vi "Refresh Modules.vi"(8 "error in (no error)":errorcluster, 11 "target address (localhost)":string="localhost") -> (0 "error out":errorcluster)   [LabVIEW 2020]
doc: "Discovers new I/O modules on any local or networked target. If a local I/O module is detected in a slot that was not previously deployed from a LabVIEW project, this VI creates new I/O variables for the I/O module."
uses:
  <resource>/objmgr/ni.var.rc
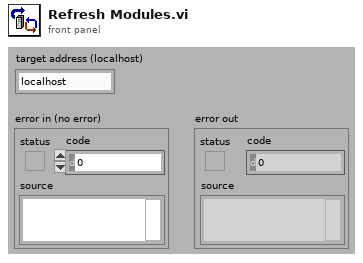
[diagram p1: front panel]
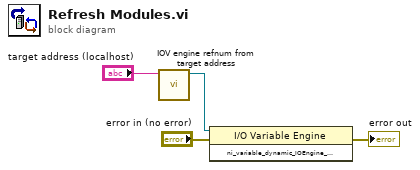
[diagram p0: block diagram]
diagram:
  n1 = call <vilib>:"IOV engine refnum from target address.vi"("target address"="target address (localhost)") -> ("reference out"=w3:refnum<k21>)  [unwired: 10 in]
  n2 = invoke class="I/O Variable Engine" method="ni_variable_dynamic_IOEngine_RefreshAutoPublished"(reference=w3, error in="error in (no error)") -> (error out=→"error out":errorcluster)  [unwired: 1 in, 2 out]
